vi "New Color.vi"(8 "error in (no error)":errorcluster, 11 "Color Box":u32(colorbox)) -> (0 "error out":errorcluster, 3 "Color out":refnum<class "Color.lvclass">)   [LabVIEW 2020, in "RPI.SenseHat.Display.lvlib" / "Color.lvclass"]
doc: "Initializes a Color object."
uses:
  Color.lvclass
  Color.lvclass/Color.ctl
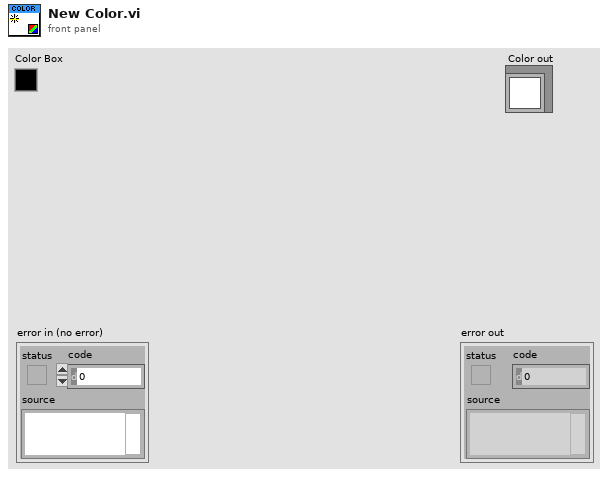
[diagram p1: front panel]
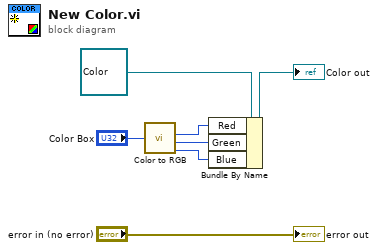
[diagram p0: block diagram]
diagram:
  n1 = call <vilib>:"Color to RGB.vi"("Color"="Color Box") -> ("R"=w3:u8, "G"=w2:u8, "B"=w1:u8)  [unwired: 1 out]
  n2 = Bundle By Name(cluster=refnum<class "Color.lvclass"> refnum ("Color in"), "Red"=w3, "Green"=w2, "Blue"=w1) -> (→"Color out":refnum<class "Color.lvclass">)
  "error out" <- "error in (no error)"
